vi "1553 Address Handles to Write Info.vi"(8 "error in":errorcluster, 11 "Address Based Execution Unit Implementation in":refnum<class "Address Based Execution Unit.lvclass">) -> (0 "error out":errorcluster, 3 "Address Based Execution Unit Implementation out":refnum<class "Address Based Execution Unit.lvclass">)   [LabVIEW 2020, in "Ballard MIL-STD-1553 Engine.lvlib" / "Implementation.lvlib" / "Address Based Execution Unit.lvclass"]
uses:
  Address Based Execution Unit.lvclass
  C:/Users/nitest/Desktop/Git 2020/niveristand-aim-milStd1553-custom-device/Source/Custom Device Support/Engine/Implementation/Execution Unit/Execution Unit.lvclass
  Address Write Info.ctl
  Shared/Address.ctl
  Acyclic Trigger Info.ctl
  Execution Unit/Execution Unit.lvclass/Execution Unit.ctl
  Address Based Execution Unit.lvclass/Address Based Execution Unit.ctl
  Execution Unit/Execution Unit.lvclass
  Custom Device/Custom Device.lvlib
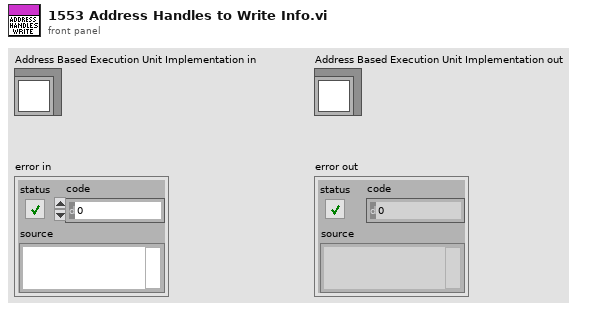
[diagram p1: front panel]
types:
  T1 = typedef "Ballard MIL-STD-1553 Engine.lvlib/Implementation.lvlib/Address Based Execution Unit.lvclass/Acyclic Trigger Info.ctl" = cluster{"bus controller handle":u64, "name":string}
  T2 = typedef "Ballard MIL-STD-1553 Engine.lvlib/Implementation.lvlib/Address Based Execution Unit.lvclass/Address Write Info.ctl" = cluster{"terminal address":T3, "terminal handle":u64}
  T3 = typedef "Address.ctl" = u16
  T4 = typedef "Ballard MIL-STD-1553 Engine.lvlib/Implementation.lvlib/Address Based Execution Unit.lvclass/1553 Address Based Handles.ctl" = cluster{"start stop handles":T5[], "acyclic frame trigger handles":T7[]}
  T5 = typedef "Ballard MIL-STD-1553 Engine.lvlib/Implementation.lvlib/Address Based Execution Unit.lvclass/Start Stop Channel Handles.ctl" = cluster{"terminal address":T3, "start handle":T6, "stop handle":T6}
  T6 = typedef "Custom Device API.lvlib/Custom Device Item Ref.ctl" = u64
  T7 = typedef "Ballard MIL-STD-1553 Engine.lvlib/Implementation.lvlib/Address Based Execution Unit.lvclass/Acyclic Frame Trigger Handle.ctl" = cluster{"name":string, "handle":T6}
  T8 = typedef "Ballard MIL-STD-1553 Engine.lvlib/Custom Device.lvlib/Hardware Handles.ctl" = cluster{"core handle":u64, "core reader handle":u64, "channel handles":u64[]}
  T9 = typedef "1553 Channel.ctl" = cluster{"HW channel":u16, "terminal addresses":T3[], "terminal names":string[], "acyclic frame names":string[], "messages":T10[]}
  T10 = typedef "Message Definition.ctl" = cluster{"name":string, "message type":T11, "endpoint Tx":T12, "endpoint Rx":T12, "create timestamp channel":bool, "mode code":u16, "number of words":u16, "parameters":cluster{"name":string, "default value":dbl, "unit":string, "parameter definition":T13}[]}
  T11 = typedef "Message Type.ctl" = string
  T12 = typedef "Terminal Endpoint.ctl" = cluster{"terminal address":T3, "subaddress":T3}
  T13 = typedef "Parameter Definition.ctl" = cluster{"start index":i32, "size (bits)":i32, "encoding":enum16{"BNR", "BCD", "Discrete"}, "signed":bool, "multiplier":dbl, "offset":dbl}
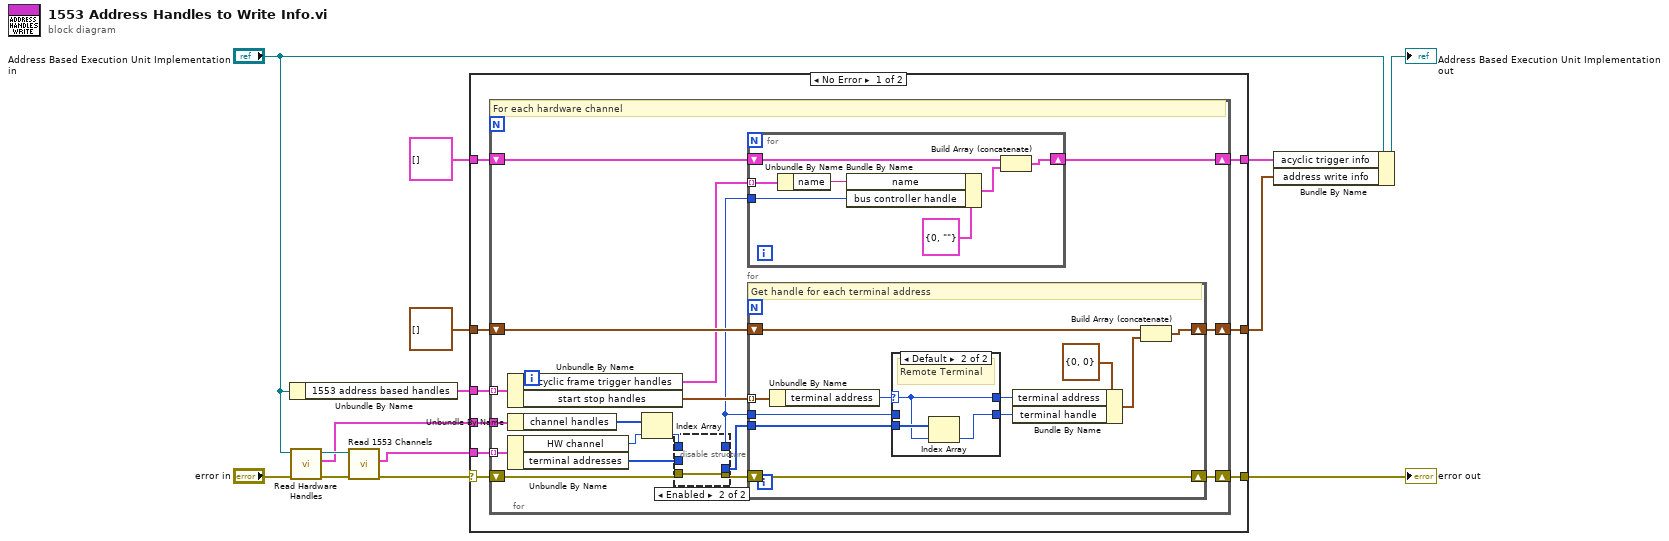
[diagram p0: block diagram]
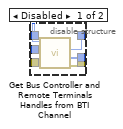
[diagram p2: hidden frame]
diagram:
  n1 = Unbundle By Name("Address Based Execution Unit Implementation in") -> ("1553 address based handles"=w6:T4[])
  n2 = call "Read Hardware Handles.vi"("error in"="error in", "Execution Unit in"="Address Based Execution Unit Implementation in") -> ("error out"=w10:errorcluster, "hardware handles"=w7:T8, "Execution Unit out"=w8:refnum<class "Address Based Execution Unit.lvclass">)  [unwired: 7 in]
  n3 = call "Read 1553 Channels.vi"("error in"=w10, "Execution Unit in"=w8) -> ("error out"=w11:errorcluster, "1553 channels"=w12:T9[])  [unwired: 7 in, 1 out]
  n4 = case shown="No Error" w11 {
    selector: w11 -> [w22 w72]
    tunnel: w12 -> [w19 _]
    tunnel: w7 -> [w23 _]
    tunnel: [w21 w72] -> w14
    tunnel: w6 -> [w20 _]
    tunnel: T2[] [] ("address write info") -> [w18 _]
    tunnel: [w17 _] -> w3
    tunnel: T1[] [] -> [w16 _]
    tunnel: [w15 _] -> w1
    frame No Error {
      n5 = for {
        tunnel: w19 -> [w41] mode=indexing
        tunnel: w23 -> [w40]
        shift-right: [w37] -> w21
        shift-left: w22 -> [w29]
        tunnel: w20 -> [w33] mode=indexing
        shift-right: [w34] -> w17
        shift-left: w18 -> [w35]
        shift-right: [w31] -> w15
        shift-left: w16 -> [w32]
        # "For each hardware channel"
        n6 = Unbundle By Name(w33) -> ("acyclic frame trigger handles"=w25:T7[], "start stop handles"=w36:T5[])
        n7 = Unbundle By Name(w40) -> ("channel handles"=w39:u64[])
        n8 = Unbundle By Name(w41) -> ("HW channel"=w38:u16, "terminal addresses"=w24:T3[])
        n9 = Index Array(array=w39, index=w38) -> (element=w30:u64)
        n10 = disable-structure shown="Enabled" {
          disable-tunnel: w30 -> [w47 _]
          disable-tunnel: w29 -> [w46 w48]
          disable-tunnel: [w45 w48] -> w28
          disable-tunnel: [w44 _] -> w27
          disable-tunnel: [w43 _] -> w26
          disable-tunnel: w24 -> [w42 _]
          frame Disabled {
            n11 = call "Get Bus Controller and Remote Terminals Handles from BTI Channel.vi"("error in"=w46, "terminal addresses"=w42, "channel handle in"=w47) -> ("error out"=w45:errorcluster, "remote terminal handles out"=w44:u64[], "bus controller handle out"=w43:u64)  [unwired: 5 in, 1 out]
          }
          frame Enabled {
          }
        }
        n12 = for {
          tunnel: w25 -> [w55] mode=indexing
          tunnel: w26 -> [w52]
          shift-right: [w50] -> w31
          shift-left: w32 -> [w53]
          n13 = Unbundle By Name(w55) -> ("name"=w49:string)
          n14 = Bundle By Name(cluster=T1 {"bus controller handle"=0, "name"=""} ("acyclic trigger info"), "name"=w49, "bus controller handle"=w52) -> (w51:T1)
          n15 = Build Array (concatenate)(w53, w51) -> (w50:T1[])
        }
        n16 = for {
          shift-right: [w66] -> w37
          shift-left: w28 -> [w66]
          tunnel: w27 -> [w64]
          tunnel: w36 -> [w65] mode=indexing
          tunnel: w26 -> [w62]
          shift-right: [w56] -> w34
          shift-left: w35 -> [w58]
          # "Get handle for each terminal address"
          n17 = Unbundle By Name(w65) -> ("terminal address"=w63:T3)
          n18 = case shown="Default" w63 {
            selector: w63 -> [w67 w69]
            tunnel: w64 -> [_ w71]
            tunnel: [w68 w70] -> w59
            tunnel: w62 -> [w68 _]
            tunnel: [w67 w69] -> w60
            frame 0 {
              # "Bus Controller"
            }
            frame Default {
              # "Remote Terminal"
              n19 = Index Array(array=w71, index=w69) -> (element=w70:u64)
            }
          }
          n20 = Bundle By Name(cluster=T2 {"terminal address"=0, "terminal handle"=0} ("address write info"), "terminal address"=w60, "terminal handle"=w59) -> (w57:T2)
          n21 = Build Array (concatenate)(w58, w57) -> (w56:T2[])
        }
      }
    }
    frame Error {
    }
  }
  "error out" <- w14
  n22 = Bundle By Name(cluster="Address Based Execution Unit Implementation in", "acyclic trigger info"=w1, "address write info"=w3) -> (→"Address Based Execution Unit Implementation out":refnum<class "Address Based Execution Unit.lvclass">)
